vi "Close DAQ.vi"(8 "error in":errorcluster, 11 "Run info":T1) -> (0 "error out":errorcluster)   [LabVIEW 2012]
uses:
  Run info.ctl
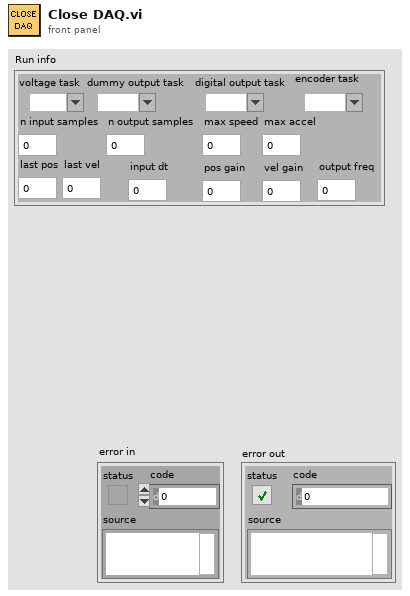
[diagram p1: front panel]
types:
  T1 = typedef "Run info.ctl" = cluster{"voltage task":refnum<k21>, "dummy output task":refnum<k21>, "digital output task":refnum<k21>, "encoder task":refnum<k21>, "n input samples":i32, "n output samples":i32, "max speed":dbl, "max accel":dbl, "last pos":dbl, "last vel":dbl, "pos gain":dbl, "vel gain":dbl, "input dt":dbl, "output freq":dbl}
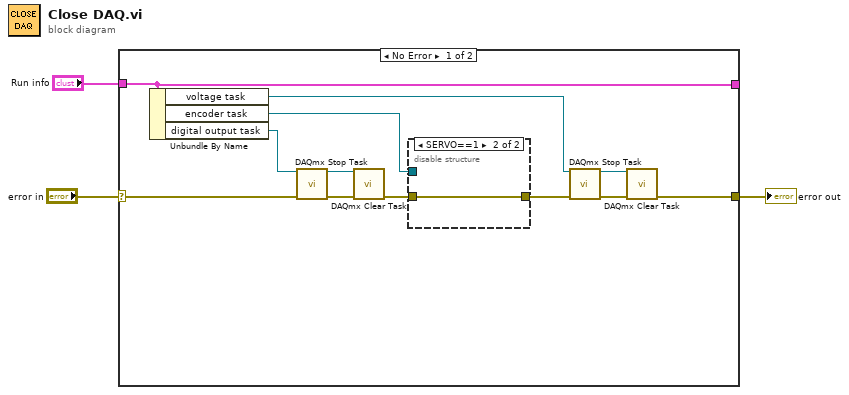
[diagram p0: block diagram]
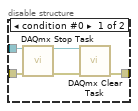
[diagram p2: hidden frame]
diagram:
  n1 = case shown="No Error" "error in" {
    selector: "error in" -> [w8 w22]
    tunnel: "Run info" -> [w15 w23]
    tunnel: [w7 w22] -> w1
    tunnel: [w15 w23] -> _
    frame No Error {
      n2 = Unbundle By Name(w15) -> ("voltage task"=w9:refnum<k21>, "encoder task"=w4:refnum<k21>, "digital output task"=w14:refnum<k21>)
      n3 = call <vilib>:"DAQmx Stop Task.vi"("task/channels in"=w14, "error in"=w8) -> ("task out"=w13:refnum<k21>, "error out"=w12:errorcluster)  [unwired: 12 in]
      n4 = call <vilib>:"DAQmx Clear Task.vi"("task in"=w13, "error in"=w12) -> ("error out"=w6:errorcluster)  [unwired: 13 in]
      n5 = disable-structure shown="SERVO==1" {
        disable-tunnel: w6 -> [w18 w21]
        disable-tunnel: [w17 w21] -> w5
        disable-tunnel: w4 -> [w16 _]
        frame condition #0 {
          n6 = call <vilib>:"DAQmx Stop Task.vi"("task/channels in"=w16, "error in"=w18) -> ("task out"=w19:refnum<k21>, "error out"=w20:errorcluster)  [unwired: 12 in]
          n7 = call <vilib>:"DAQmx Clear Task.vi"("task in"=w19, "error in"=w20) -> ("error out"=w17:errorcluster)  [unwired: 13 in]
        }
        frame condition #1 (active) {
        }
      }
      n8 = call <vilib>:"DAQmx Stop Task.vi"("task/channels in"=w9, "error in"=w5) -> ("task out"=w10:refnum<k21>, "error out"=w11:errorcluster)  [unwired: 12 in]
      n9 = call <vilib>:"DAQmx Clear Task.vi"("task in"=w10, "error in"=w11) -> ("error out"=w7:errorcluster)  [unwired: 13 in]
    }
    frame Error {
    }
  }
  "error out" <- w1
